vi "KR_Module.vi"() -> ()   [LabVIEW 2012]
doc: "SciScan 1.2 160630"
uses:
  Custom Control and Typedefs/ChannelSelector_for_PosSave.ctl
  Custom Control and Typedefs/Overlay Control.ctl
  Custom Control and Typedefs/UI Controls Refnum.ctl
  <vilib>/vision/Image Controls.llb/IMAQ Image.ctl
  SubVIs/Chnl_2_tab_Commands.ctl
  SubVIs/Image Validity FGV_Commands.ctl
  Custom Controls/MAIN Image panel tab Control type def.ctl
  CommonResource VIs/UI Control and Indicator properties_Commands.ctl
  Custom Control and Typedefs/ImageCluster.ctl
  GFG/GFG library.lvlib
  Libtiff3/libtiff3.llb/libtiff3.lvlib
panel:
  out "x-y":u32
  in  "Pop-Out 2":bool caption="Pop-Out"
  in  "Pop-Out":bool
  in  "no of grid lines 2":dbl(slide)=2.0 caption="Grid" min=0.0 step=1.0 scale=0.0..20.0
  in  "FOCUS2":bool
  in  "Overlay Controls":T1={"auto scale\n      Red "=TRUE, "Min Max Saved (Green)"={0.0, 1618.0}, "auto scale\n      Green"=TRUE, "Min Max Saved (Red)"={0.0, 1618.0}} {"Min Max Saved (Red)" scale=-32768.0..32767.0; "Min Max Saved (Green)" scale=-32768.0..32767.0}
  in  "File Path":path
  in  "Overlay":bool
  in  "Source":T2
  out "Saved Image":T3(plugin-control)
  out "Current Image":T3(plugin-control)
  # "Red (Current Image)"
  # "Green (Saved Image)"
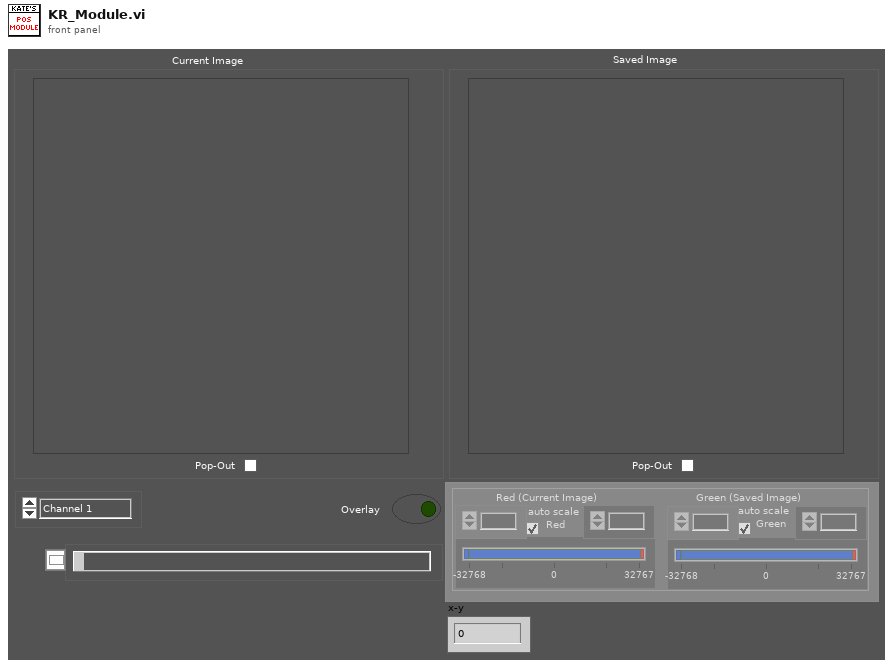
[diagram p1: front panel]
types:
  T1 = typedef "Overlay Control.ctl" = cluster{"auto scale\n      Red ":bool, "Min Max Saved (Green)":cluster{dbl, dbl}, "auto scale\n      Green":bool, "Min Max Saved (Red)":cluster{dbl, dbl}}
  T2 = typedef "ChannelSelector_for_PosSave.ctl" = enum16{"Channel 1", "Channel 2", "Channel 3", "Channel 4"}
  T3 = typedef "IMAQ Image.ctl" = refnum<image>
  T4 = typedef "Image Type" = u32
  T5 = typedef "UI Controls Refnum.ctl" = cluster{"GO TO":refnum<vi>, "Load List":refnum<vi>, "Big Table":refnum<vi>, "Notes Table":refnum<vi>, "New List":refnum<vi>, "Delete Item":refnum<vi>, "Set New Origin":refnum<vi>, "Set POI":refnum<vi>, "Saved Image":refnum<vi>, "Current Image":refnum<vi>, "step.size.xy 2":refnum<vi>, "step.size.z 2":refnum<vi>, "Source":refnum<vi>, "Table Up-End":refnum<vi>, "Table Up":refnum<vi>, "Table Down":refnum<vi>, "Table Down-End":refnum<vi>, "Copy Button":refnum<vi>, "Hide":refnum<vi>, "Overlay Controls":refnum<vi>, "Overlay":refnum<vi>, "XYGraph":refnum<vi>, "FOCUS2":refnum<vi>}
  T6 = enum8{"Enabled", "Disabled", "Disabled and Grayed Out"}
  T7 = typedef "ImageCluster.ctl" = cluster{"CurrentImage":T3, "SavedImage":T3}
  T8 = enum32{"Invalid", "Standard", "Closed", "Hidden", "Minimized", "Maximized"}
  T9 = typedef "Image Validity FGV_Commands.ctl" = enum16{"Set validity status", "Get Validity status"}
  T10 = typedef "Chnl_2_tab_Commands.ctl" = enum16{"ChannelToTab", "TabToChannel"}
  T11 = typedef "MAIN Image panel tab Control type def.ctl" = enum32{"Channel 1", "Channel 2", "Channel 3", "Channel 4", "all channels", "RGB overlay", "ROI", "arbitrary line scan"}
  T12 = typedef "UI Control and Indicator properties_Commands.ctl" = enum16{"Enable", "Disable", "Disable and Grey", "Make Visible", "Make Invisible"}
  T13 = cluster{"WaveformChartRef":refnum<vi>, "DigitalRef":refnum<vi>, "ArrayRef":refnum<vi>, "TabControlRef":refnum<vi>, "EnumRef":refnum<vi>, "RingRef":refnum<vi>, "BooleanRef":refnum<vi>, "KnobRef":refnum<vi>, "SlideRef":refnum<vi>, "PathRef":refnum<vi>, "StringRef":refnum<vi>, "ComboBox":refnum<vi>, "WaveformGraphRef":refnum<vi>}
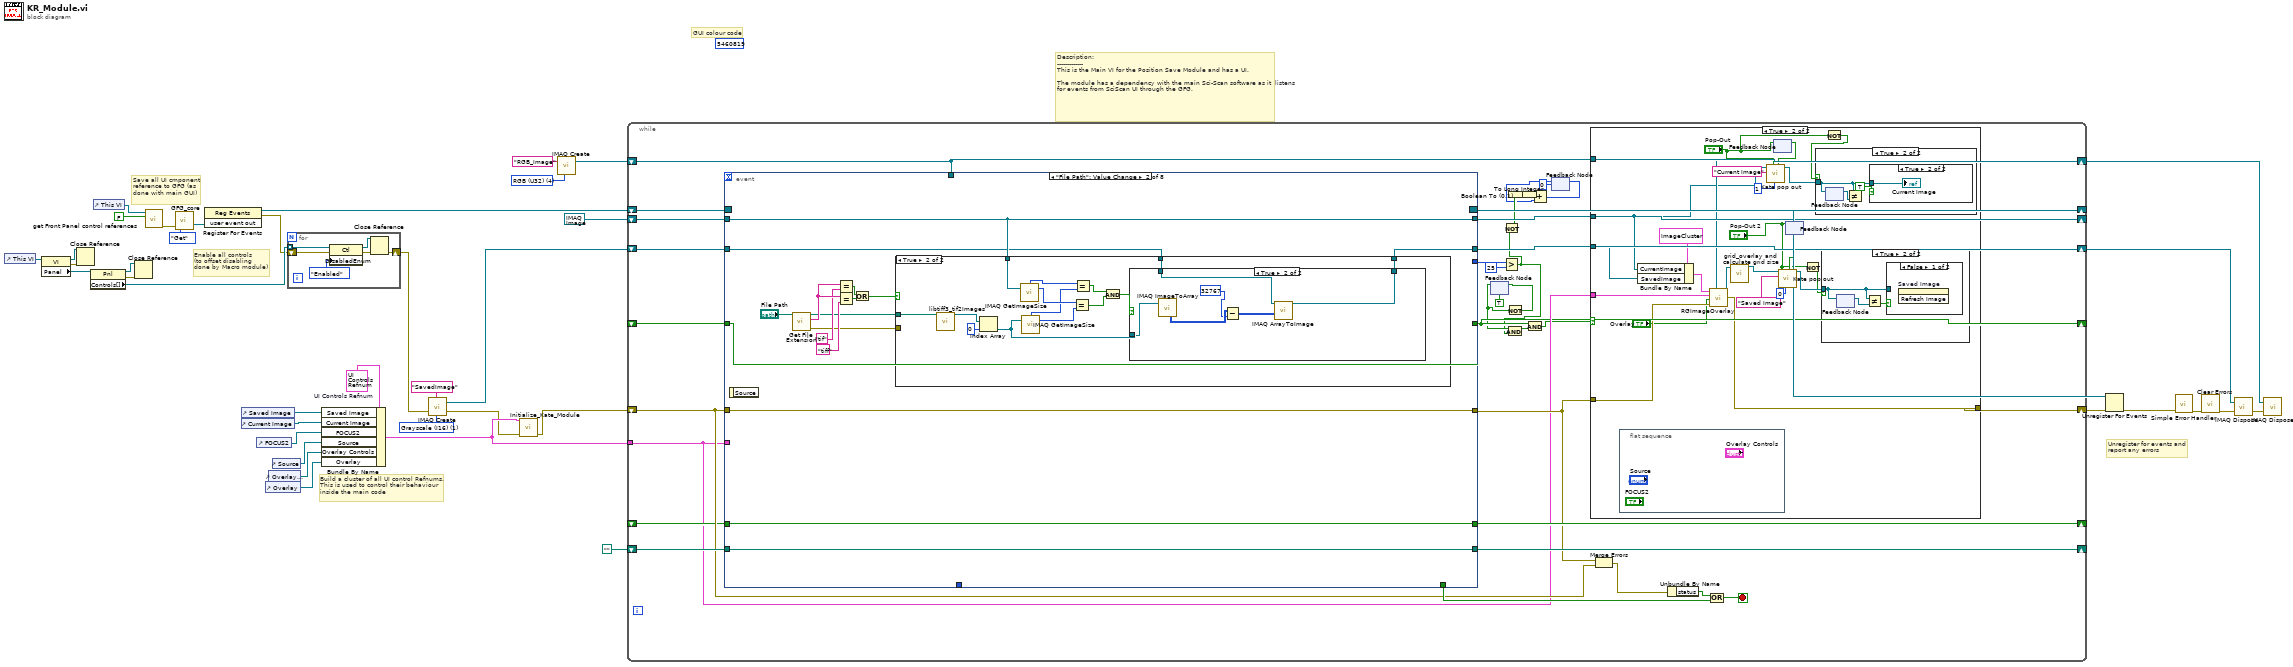
[diagram p0: block diagram]
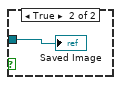
[diagram p4: hidden frame]
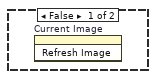
[diagram p6: hidden frame]
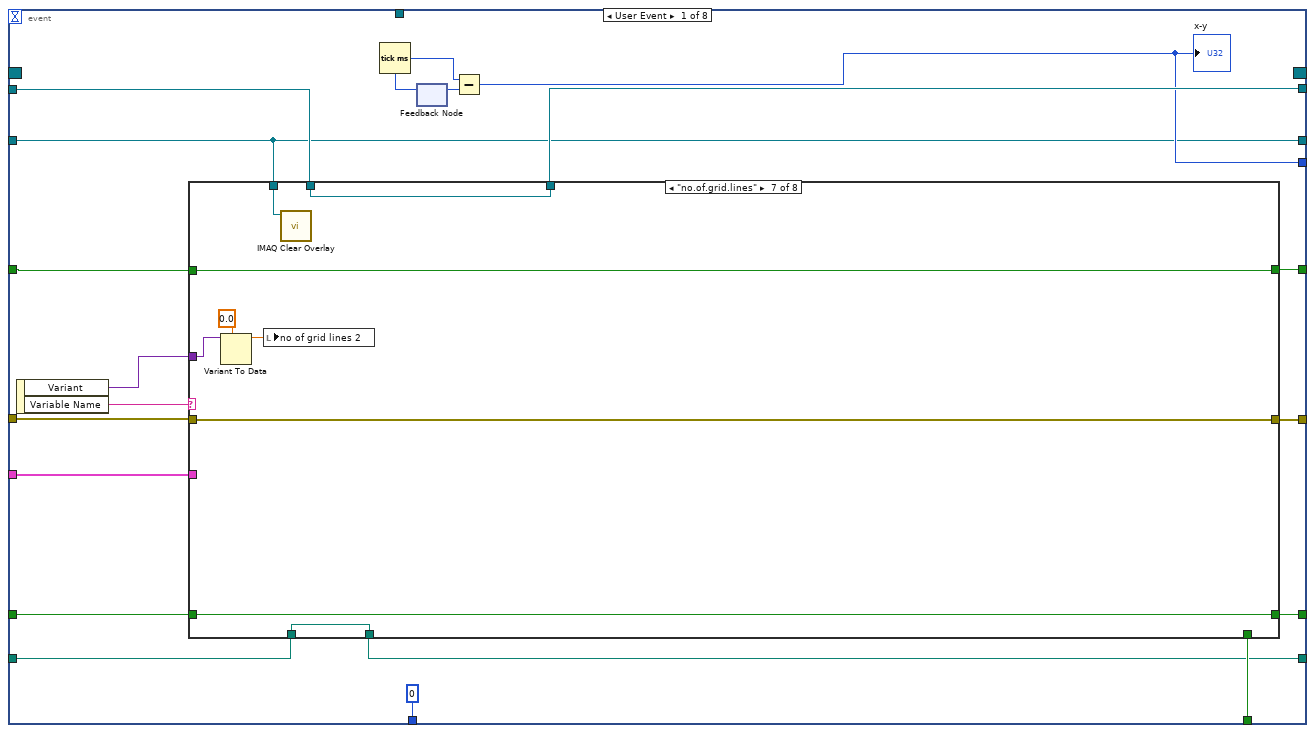
[diagram p7: hidden frame]
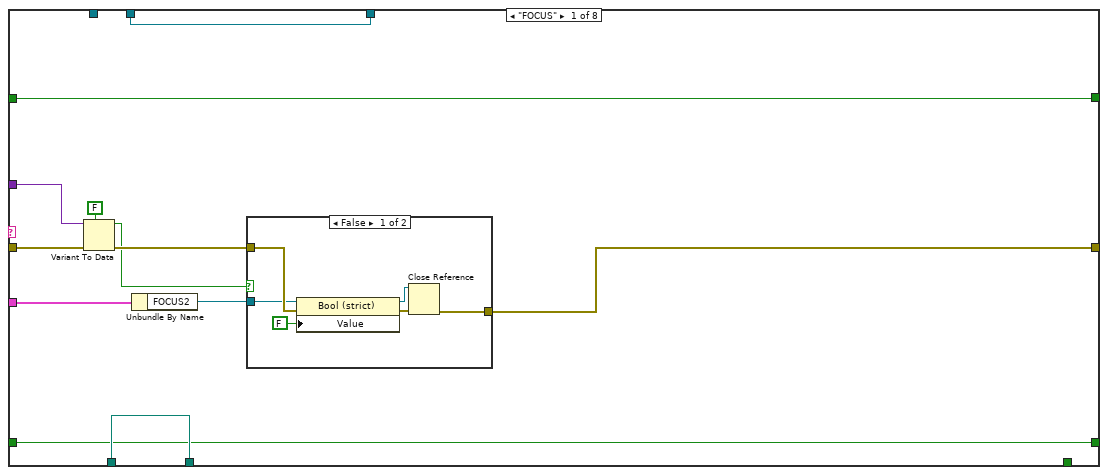
[diagram p8: hidden frame]
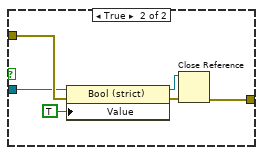
[diagram p9: hidden frame]
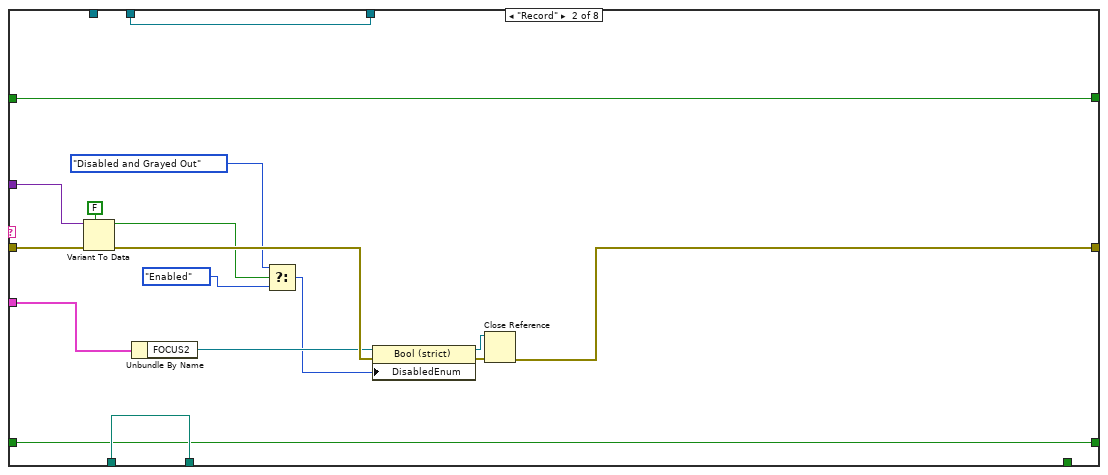
[diagram p10: hidden frame]
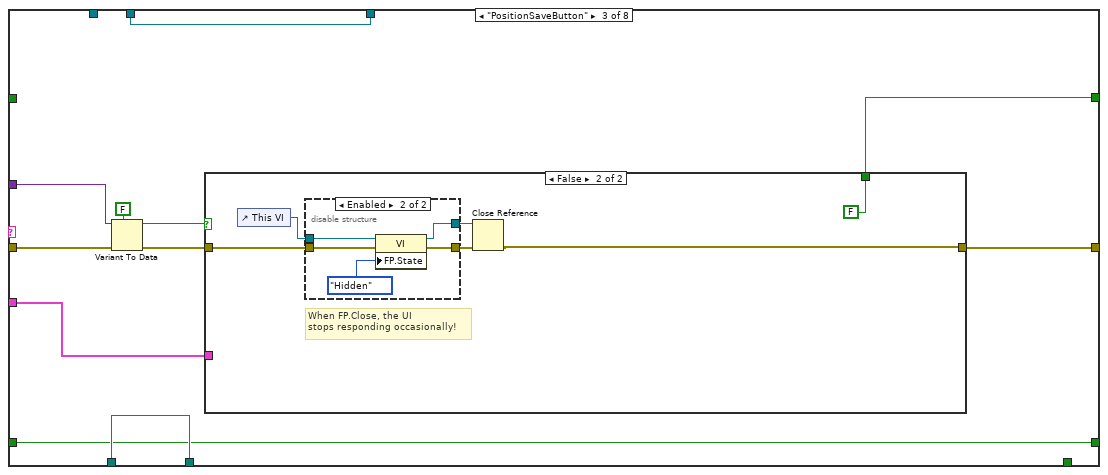
[diagram p11: hidden frame]
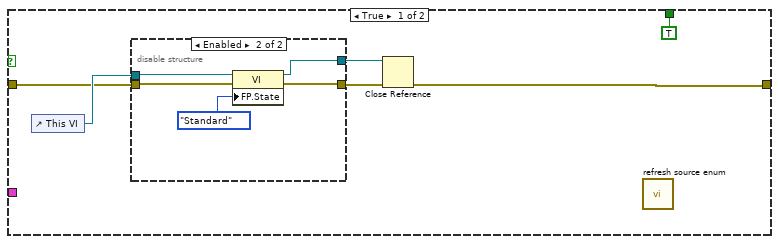
[diagram p12: hidden frame]
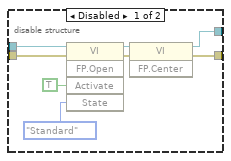
[diagram p13: hidden frame]
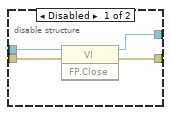
[diagram p14: hidden frame]
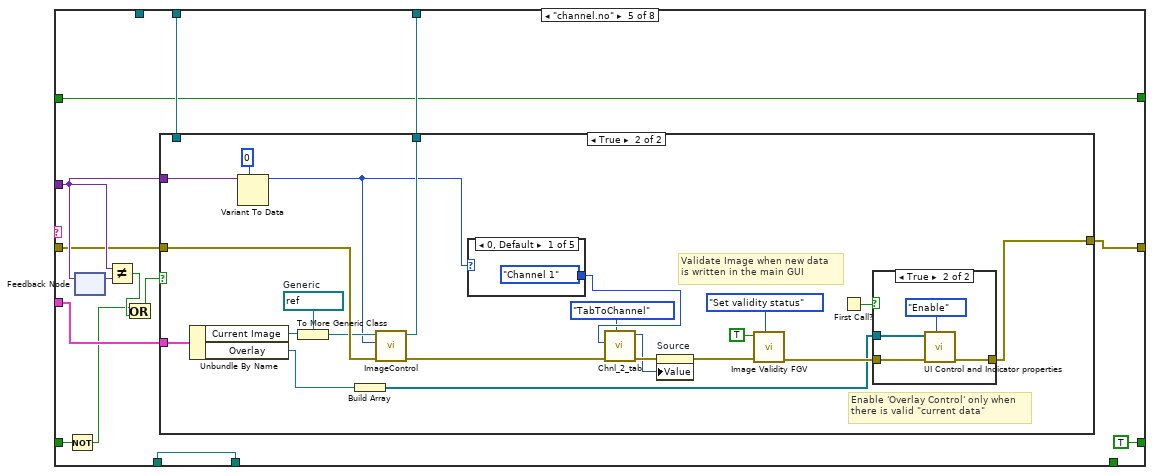
[diagram p16: hidden frame]
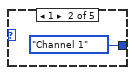
[diagram p18: hidden frame]
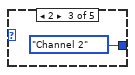
[diagram p19: hidden frame]
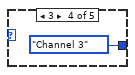
[diagram p20: hidden frame]
diagram:
  w25 = T4 4 items=["Grayscale (U8)", "Grayscale (I16)", "Grayscale (SGL)", "Complex (CSG)", "RGB (U32)", "HSL (U32)", "RGB (U64)", "Grayscale (U16)"] ("Image Type")
  w31 = T4 1 items=["Grayscale (U8)", "Grayscale (I16)", "Grayscale (SGL)", "Complex (CSG)", "RGB (U32)", "HSL (U32)", "RGB (U64)", "Grayscale (U16)"] ("Image Type")
  (unwired) u32 5460819 ("Active Cell:Cell Background Color")
  w37 = T5 {"GO TO"=refnum, "Load List"=refnum, "Big Table"=refnum, "Notes Table"=refnum, "New List"=refnum, "Delete Item"=refnum, "Set New Origin"=refnum, "Set POI"=refnum, "Saved Image"=refnum, "Current Image"=refnum, "step.size.xy 2"=refnum, "step.size.z 2"=refnum, "Source"=refnum, "Table Up-End"=refnum, "Table Up"=refnum, "Table Down"=refnum, "Table Down-End"=refnum, "Copy Button"=refnum, "Hide"=refnum, "Overlay Controls"=refnum, "Overlay"=refnum, "XYGraph"=refnum, "FOCUS2"=refnum}  # UI Controls Refnum
  # "Enable all controls\n(to offset disabling \ndone by Macro module)"
  # "GUI colour code"
  # "Save all UI cmponent reference to GFG (as done with main GUI)"
  # "Build a cluster of all UI control Refnums.\nThis is used to control their behaviour \ninside the main code"
  # "Unregister for events and \nreport any errors"
  # "Description:\n-------------\nThis is the Main VI for the Position Save Module and has a UI.\n\nThe module has a dependency with the main Sci-Scan software as it  listens for events from SciScan UI through the GFG."
  n1 = control-ref of="This VI"() -> (w17:refnum<vi>)
  n2 = property class="VI"(reference=w17) -> (reference out=w14:refnum<vi>, error out=w15:errorcluster, "Panel"=w16:refnum<vi>)  [unwired: 1 in]
  n3 = Close Reference(reference=w14, error in (no error)=w15) -> ()  [unwired: 1 out]
  n4 = property class="Pnl"(reference=w16) -> (reference out=w12:refnum<vi>, error out=w13:errorcluster, "Controls[]"=w11:refnum<vi>[])  [unwired: 1 in]
  n5 = control-ref of="This VI"() -> (w36:refnum<vi>)
  n6 = Close Reference(reference=w12, error in (no error)=w13) -> ()  [unwired: 1 out]
  n7 = call "get Front Panel control references.vi"("Signalling (Default: T)"=FALSE, "Main VI"=w36) -> ("error out"=w8:errorcluster)  [unwired: 9 in]
  n8 = call "GFG_core.vi"("error in (no error)"=w8, "Action"=enum16{"Init", "Set", "Get"}."Get") -> ("user event out"=w39:refnum<user-event>)  [unwired: 11 in, 6 out]
  n9 = register-events(w39) -> (reference out=w40:refnum<event-registration>, error out=w10:errorcluster)  [unwired: 2 in]
  n10 = control-ref of="Saved Image"() -> (w34:refnum<vi>)
  n11 = control-ref of="Current Image"() -> (w33:refnum<vi>)
  n12 = control-ref of="FOCUS2"() -> (w7:refnum<vi>)
  n13 = control-ref of="Overlay"() -> (w5:refnum<vi>)
  n14 = control-ref of="Overlay Controls"() -> (w4:refnum<vi>)
  n15 = control-ref of="Source"() -> (w6:refnum<vi>)
  n16 = for {
    tunnel: w11 -> [w47] mode=indexing
    shift-right: [w43] -> w9
    shift-left: w10 -> [w42]
    n17 = property class="Ctl"(reference=w47, error in=w42, "DisabledEnum"=T6."Enabled" ("Disabled")) -> (reference out=w44:refnum<vi>, error out=w45:errorcluster)
    n18 = Close Reference(reference=w44, error in (no error)=w45) -> (error out=w43:errorcluster)
  }
  n19 = Bundle By Name(cluster=w37, "Saved Image"=w34, "Current Image"=w33, "FOCUS2"=w7, "Source"=w6, "Overlay Controls"=w4, "Overlay"=w5) -> (w3:T5)
  n20 = call "IMAQ Create"("Image Name"="SavedImage", "Image Type"=w31, "error in (no error)"=w9) -> ("New Image"=w30:T3, "error out"=w2:errorcluster)  [unwired: 2 in]
  n21 = call "Initialize_Kate_Module.vi"("Error In"=w2, "UI Controls Refnum"=w3) -> ("Error Out"=w1:errorcluster)  [unwired: 9 in]
  n22 = call "IMAQ Create"("Image Name"="RGB_Image", "Image Type"=w25) -> ("New Image"=w24:T3)  [unwired: 3 in, 1 out]
  n23 = while {
    shift-right: [w67] -> w28
    shift-left: w1 -> [w74]
    shift-right: [w78] -> w38
    shift-left: w40 -> [w79]
    tunnel: w3 -> [w66]
    shift-right: [w64] -> _
    shift-left: T3 refnum ("Saved Image OUT") -> [w77]
    shift-right: [w72] -> w20
    shift-left: w30 -> [w76]
    shift-right: [w69] -> _
    shift-left: path "" -> [w75]
    shift-right: [w65] -> w19
    shift-left: w24 -> [w65]
    shift-right: [w71] -> _
    shift-left: _ -> [w70]
    shift-right: [w61] -> _
    shift-left: _ -> [w63]
    stop <- w80 stop-if-true
    n24 = event shown="[1] \"File Path\": Value Change" {
      selector: w79 -> [_ _ _ _ _ _ _ _]
      dyn-events: [_ _ _ _ _ _ _ _] -> w78
      timeout: _ -> [_ _ _ _ _ _ _ _]
      tunnel: [w133 _ _ _ _ _ _ _] -> w82
      tunnel: w74 -> [w132 w332 w362 w383 w403 w426 w448 w460]
      tunnel: [w131 w332 w361 w382 w403 w413 w445 w460] -> w68
      tunnel: w66 -> [w129 _ _ w385 _ _ _ _]
      tunnel: [w128 w329 w378 w389 w406 w423 w456 w463] -> w64
      tunnel: w77 -> [w125 w329 w378 w389 w406 w423 w456 w463]
      tunnel: [w115 w327 w377 w388 w405 w422 w455 w458] -> w72
      tunnel: w76 -> [w115 w328 w377 w388 w405 w422 w455 w462]
      tunnel: [w126 w331 w375 w387 w404 w418 w454 w459] -> w69
      tunnel: w75 -> [w127 w331 w375 w387 w404 w418 w454 w459]
      tunnel: [0 ("x-y 2") _ _ 1 ("x-y 2") 2 ("x-y 2") 17 ("x-y 2") 19 ("x-y 2") _] -> _
      tunnel: [w122 w330 w360 w380 w401 w408 w443 w461] -> w71
      tunnel: w70 -> [w121 w330 w360 w380 w401 w408 w443 w461]
      tunnel: w65 -> [_ _ _ _ _ _ _ _]
      tunnel: [w120 w326 w359 w379 w400 w407 w442 w457] -> w61
      tunnel: w63 -> [w119 w326 w359 w379 w400 w407 w442 w457]
      tunnel: [w116 _ _ _ _ _ _ _] -> w56
      event User Event {
        n25 = event-data() -> ("Variant"=w130:variant, "Variable Name"=w123:string)  [unwired: 1 in]
        n26 = case shown="\"no.of.grid.lines\"" w123 {
          tunnel: [_ _ _ _ _ _ _ TRUE] -> w133
          tunnel: w132 -> [w142 w171 w185 w222 w235 w284 w307 w312]
          tunnel: [w138 w168 w180 w222 w232 w281 w307 w312] -> w131
          tunnel: w130 -> [w140 w169 w183 _ w237 w287 w306 _]
          tunnel: [w144 w173 w177 w224 w234 w285 w310 w315] -> w128
          tunnel: w129 -> [w137 w167 w178 _ w233 w283 _ _]
          tunnel: w127 -> [w145 w174 w179 w223 w238 w286 w309 _]
          tunnel: [w145 w174 w179 w223 w238 w286 w309 path ""] -> w126
          tunnel: w125 -> [w144 w173 w177 w224 w226 w285 w310 w315]
          tunnel: [w135 w165 w176 w221 TRUE ("Validity status IN") w274 w308 w314] -> w122
          tunnel: w121 -> [w135 w165 w176 w221 w228 w274 w308 w314]
          tunnel: [w134 w158 w175 w220 w225 w273 w303 w311] -> w120
          tunnel: w119 -> [w134 w158 _ w220 w225 w273 w303 w311]
          tunnel: w115 -> [_ _ _ _ _ _ w302 _]
          frame "FOCUS" {
            n27 = Variant To Data(error in=w142, type=FALSE ("Value"), Variant=w140) -> (data=w139:bool, error out=w141:errorcluster)
            n28 = Unbundle By Name(w137) -> ("FOCUS2"=w136:refnum<vi>)
            n29 = case shown="False" w139 {
              tunnel: w141 -> [w150 w156]
              tunnel: [w147 w153] -> w138
              tunnel: w136 -> [w146 w152]
              frame False {
                n30 = property class="Bool (strict)"(reference=w146, error in=w150, "Value"=FALSE) -> (reference out=w148:refnum<vi>, error out=w149:errorcluster)
                n31 = Close Reference(reference=w148, error in (no error)=w149) -> (error out=w147:errorcluster)
              }
              frame True {
                n32 = property class="Bool (strict)"(reference=w152, error in=w156, "Value"=TRUE) -> (reference out=w154:refnum<vi>, error out=w155:errorcluster)
                n33 = Close Reference(reference=w154, error in (no error)=w155) -> (error out=w153:errorcluster)
              }
            }
          }
          frame "Record" {
            n34 = Variant To Data(error in=w171, type=FALSE ("Value"), Variant=w169) -> (data=w164:bool, error out=w170:errorcluster)
            n35 = Unbundle By Name(w167) -> ("FOCUS2"=w166:refnum<vi>)
            n36 = Select(t=T6."Disabled and Grayed Out" ("Disabled"), s=w164, f=T6."Enabled" ("Disabled")) -> (s? t:f=w159:T6)
            n37 = property class="Bool (strict)"(reference=w166, error in=w170, "DisabledEnum"=w159) -> (reference out=w162:refnum<vi>, error out=w163:errorcluster)
            n38 = Close Reference(reference=w162, error in (no error)=w163) -> (error out=w168:errorcluster)
          }
          frame "PositionSaveButton" {
            n39 = Variant To Data(error in=w185, type=FALSE, Variant=w183) -> (data=w181:bool, error out=w182:errorcluster)
            n40 = case shown="False" w181 {
              tunnel: w182 -> [w190 w209]
              tunnel: [w187 w206] -> w180
              tunnel: w178 -> [_ _]
              tunnel: [TRUE FALSE] -> w175
              frame True {
                n41 = control-ref of="This VI"() -> (w191:refnum<vi>)
                n42 = disable-structure shown="Enabled" {
                  disable-tunnel: w191 -> [w199 w203]
                  disable-tunnel: w190 -> [w198 w202]
                  disable-tunnel: [w193 w201] -> w189
                  disable-tunnel: [w192 w200] -> w188
                  frame Disabled {
                    n43 = invoke class="VI" method="FP.Open"(reference=w199, error in=w198, "Activate"=TRUE ("Activate?"), "State"=T8."Standard") -> (reference out=w195:refnum<vi>, error out=w194:errorcluster)  [unwired: 1 in, 3 out]
                    n44 = invoke class="VI" method="FP.Center"(reference=w195, error in=w194) -> (reference out=w192:refnum<vi>, error out=w193:errorcluster)  [unwired: 1 in, 1 out]
                  }
                  frame Enabled {
                    n45 = property class="VI"(reference=w203, error in=w202, "FP.State"=T8."Standard" ("Front Panel Window:State")) -> (reference out=w200:refnum<vi>, error out=w201:errorcluster)
                  }
                }
                n46 = Close Reference(reference=w188, error in (no error)=w189) -> (error out=w187:errorcluster)
                n47 = call "refresh source enum.vi"() -> ()  [unwired: 12 in]
              }
              frame False {
                # "When FP.Close, the UI\nstops responding occasionally!"
                n48 = control-ref of="This VI"() -> (w210:refnum<vi>)
                n49 = disable-structure shown="Enabled" {
                  disable-tunnel: w210 -> [w214 w217]
                  disable-tunnel: w209 -> [w213 w218]
                  disable-tunnel: [w212 w219] -> w208
                  disable-tunnel: [w211 w215] -> w207
                  frame Disabled {
                    n50 = invoke class="VI" method="FP.Close"(reference=w214, error in=w213) -> (reference out=w211:refnum<vi>, error out=w212:errorcluster)  [unwired: 1 in, 1 out]
                  }
                  frame Enabled {
                    n51 = property class="VI"(reference=w217, error in=w218, "FP.State"=T8."Hidden" ("Front Panel Window:State")) -> (reference out=w215:refnum<vi>, error out=w219:errorcluster)
                  }
                }
                n52 = Close Reference(reference=w207, error in (no error)=w208) -> (error out=w206:errorcluster)
              }
            }
          }
          frame Default {
          }
          frame "channel.no" {
            n53 = Not(x=w228) -> (.not. x?=w227:bool)
            n54 = feedback #1() -> (w236:variant)  [unwired: 1 in]
            n55 = feedback-in #1(w237) -> ()
            n56 = Not Equal?(x=w237, y=w236) -> (x != y?=w230:bool)
            n57 = Or(x=w227, y=w230) -> (x .or. y?=w229:bool)
            n58 = case shown="True" w229 {
              tunnel: w237 -> [_ w262]
              tunnel: w235 -> [w239 w261]
              tunnel: [w240 w260] -> w234
              tunnel: w233 -> [_ w259]
              tunnel: [w239 w258] -> w232
              tunnel: w226 -> [w240 _]
              frame False {
              }
              frame True {
                w248 = refnum<vi> refnum  # Generic
                # "Enable 'Overlay Control' only when there is valid \"current data\""
                # "Validate Image when new data\nis written in the main GUI"
                n59 = Unbundle By Name(w259) -> ("Current Image"=w251:refnum<vi>, "Overlay"=w250:refnum<vi>)
                n60 = Variant To Data(type=0, Variant=w262) -> (data=w247:i32)  [unwired: 1 in, 1 out]
                n61 = To More Generic Class(target class=w248, reference=w251) -> (generic class reference=w252:refnum<vi>)
                n62 = Build Array(w250) -> (w249:refnum<vi>[])
                n63 = call "ImageControl.vi"("Error In"=w261, "Channel No"=w247, "Image Refnum (Generic)"=w252) -> ("Error Out"=w253:errorcluster, "Current Image"=w260:T3)  [unwired: 7 in]
                n64 = case shown="0, Default" w247 {
                  tunnel: [MAIN_Image_panel_tab_Control_type_def."Channel 1" ("Tab IN") MAIN_Image_panel_tab_Control_type_def."Channel 1" ("Tab IN") MAIN_Image_panel_tab_Control_type_def."Channel 2" ("Tab IN") MAIN_Image_panel_tab_Control_type_def."Channel 3" ("Tab IN") MAIN_Image_panel_tab_Control_type_def."Channel 4" ("Tab IN")] -> w245
                  frame 0, Default {
                  }
                  frame 1 {
                  }
                  frame 2 {
                  }
                  frame 3 {
                  }
                  frame 4 {
                  }
                }
                n65 = call "Chnl_2_tab.vi"("Command"=Chnl_2_tab_Commands."TabToChannel", "Error In"=w253, "Tab IN"=w245) -> ("Error Out"=w255:errorcluster, "Channel  OUT"=w254:T2)  [unwired: 6 in, 1 out]
                n66 = property on="Source" class="Enum (strict)"(error in=w255, "Value"=w254) -> (error out=w256:errorcluster)  [unwired: 1 in, 1 out]
                n67 = call "Image Validity FGV.vi"("Image Validity FGV_Commands"=Image_Validity_FGV_Commands."Set validity status", "Error In"=w256, "Validity status IN"=TRUE) -> ("Error Out"=w257:errorcluster)  [unwired: 7 in, 1 out]
                n68 = First Call?() -> (First Call?: T/F=w241:bool)
                n69 = case shown="True" w241 {
                  tunnel: w257 -> [w268 w271]
                  tunnel: [w268 w270] -> w258
                  tunnel: w249 -> [_ w269]
                  frame False {
                  }
                  frame True {
                    n70 = call "UI Control and Indicator properties.vi"("Enable Command"=UI_Control_and_Indicator_properties_Commands."Enable", "Error In"=w271, "Control Refnums"=w269) -> ("Error Out"=w270:errorcluster)  [unwired: 8 in]
                  }
                }
              }
            }
          }
          frame "MAIN.Image.panels.", "MAIN.Image.panels.reso." {
            # "Clear Error  91 if it occurs. Eg. when \nGFG variable for the 'main image panel' of the wrong  type is set - This is triggered by MACRO MODULE"
            n71 = Unbundle By Name(w283) -> ("Source"=w282:refnum<vi>)
            n72 = Variant To Data(error in=w284, type=0, Variant=w287) -> (data=w279:i32, error out=w277:errorcluster)
            n73 = call "Clear Specific Errors.vi"("Error In"=w277, "Error number In"=91) -> ("Error Out"=w276:errorcluster, "Error Cleared?"=w275:bool)  [unwired: 8 in]
            n74 = case shown="True" w275 {
              tunnel: w282 -> [w293 _]
              tunnel: [w292 w301] -> w281
              tunnel: w279 -> [w290 _]
              tunnel: w276 -> [w288 w301]
              frame False {
                n75 = Less?(x=w290, y=4) -> (x < y?=w291:bool)
                n76 = case shown="True" w291 {
                  tunnel: w293 -> [_ w300]
                  tunnel: [w294 w297] -> w292
                  tunnel: w290 -> [_ w296]
                  tunnel: w288 -> [w294 w295]
                  frame False {
                  }
                  frame True {
                    n77 = property class="Enum (strict)"(reference=w300, error in=w295, "Value"=w296) -> (reference out=w298:refnum<vi>, error out=w299:errorcluster)
                    n78 = Close Reference(reference=w298, error in (no error)=w299) -> (error out=w297:errorcluster)
                  }
                }
              }
              frame True {
                # "Error 91 has been cleared.\nWrong 'Image Panels GFG variable' set.\nDO NOTHING!"
              }
            }
          }
          frame "no.of.grid.lines" {
            n79 = Variant To Data(type=0.0 ("no of grid lines 2"), Variant=w306) -> (data=w304:dbl)  [unwired: 1 in, 1 out]
            n80 = local write "no of grid lines 2"(w304) -> ()
            n81 = call "IMAQ Clear Overlay"("Image"=w302) -> ()  [unwired: 9 in, 2 out]
          }
          frame "QUIT" {
          }
        }
        n82 = Tick Count (ms)() -> (millisecond timer value=w118:u32)
        n83 = feedback-in #2(w118) -> ()
        n84 = feedback #2() -> (w117:u32)  [unwired: 1 in]
        n85 = Subtract(x=w118, y=w117) -> (x-y=w116:u32)
        "x-y" <- w116
      }
      event "File Path": Value Change {
        n86 = event-data() -> ()  [unwired: 1 in, 1 out]
        n87 = call <vilib>:"Get File Extension.vi"("file"="File Path") -> ("error out"=w317:errorcluster, "lowercase file extension"=w325:string, "dup file"=w318:path)  [unwired: 7 in, 1 out]
        n88 = Equal?(x=w325, y="tif") -> (x = y?=w322:bool)
        n89 = Equal?(x=w325, y="tiff") -> (x = y?=w321:bool)
        n90 = Or(x=w322, y=w321) -> (x .or. y?=w319:bool)
        n91 = case shown="True" w319 {
          tunnel: w329 -> [_ w350]
          tunnel: w328 -> [w333 w342]
          tunnel: [w333 w341] -> w327
          tunnel: w318 -> [_ w338]
          tunnel: w317 -> [w335 _]
          frame False {
            # "Ignore this file, as it's not a TIFF."
            n92 = property on="File Path" class="Path"(error in=w335, "Value"=path "" ("File Path")) -> ()  [unwired: 1 in, 2 out]
            n93 = One Button Dialog(message="Invalid file format! Please select a TIFF file and try again.") -> ()  [unwired: 1 in, 1 out]
          }
          frame True {
            n94 = call "libtiff3_tif2Images.vi"("Input path"=w338) -> ("ImageArray"=w340:T3[])  [unwired: 9 in, 1 out]
            n95 = Index Array(array=w340, index=0) -> (element=w337:T3)
            n96 = call "IMAQ GetImageSize"("Image"=w350) -> ("Y Resolution"=w349:i32, "X Resolution"=w346:i32)  [unwired: 3 in, 1 out]
            n97 = call "IMAQ GetImageSize"("Image"=w337) -> ("Y Resolution"=w348:i32, "X Resolution"=w347:i32)  [unwired: 3 in, 1 out]
            n98 = Equal?(x=w349, y=w348) -> (x = y?=w344:bool)
            n99 = Equal?(x=w346, y=w347) -> (x = y?=w345:bool)
            n100 = And(x=w345, y=w344) -> (x .and. y?=w343:bool)
            n101 = case shown="True" w343 {
              tunnel: w337 -> [_ w358]
              tunnel: w342 -> [w352 w354]
              tunnel: [w352 w353] -> w341
              frame False {
                n102 = One Button Dialog(message="Image Size Mismatch") -> ()  [unwired: 1 in, 1 out]
              }
              frame True {
                n103 = call "IMAQ ImageToArray"("Image"=w358) -> ("Image Pixels (U16)"=w357:u16[][])  [unwired: 3 in, 4 out]
                n104 = Subtract(x=w357, y=i16 32767) -> (x-y=w355:u16[][])
                n105 = call "IMAQ ArrayToImage"("Image Pixels (I16)"=w355, "Image"=w354) -> ("Image Out"=w353:T3)  [unwired: 8 in, 1 out]
              }
            }
          }
        }
      }
      event Panel Close? {
        n106 = event-data() -> ()  [unwired: 1 in, 1 out]
        n107 = control-ref of="This VI"() -> (w374:refnum<vi>)
        n108 = property class="VI"(reference=w374, error in=w362, "FP.State"=T8."Hidden" ("Front Panel Window:State")) -> (reference out=w372:refnum<vi>, error out=w373:errorcluster)
        n109 = Close Reference(reference=w372, error in (no error)=w373) -> (error out=w365:errorcluster)
        n110 = call "GFGfpRefGet.vi"("error in (no error)"=w365, "Variable Name in"="PositionSaveButton") -> ("error out"=w369:errorcluster, "output cluster"=w370:T13)  [unwired: 8 in]
        n111 = Unbundle By Name(w370) -> ("BooleanRef"=w368:refnum<vi>)
        n112 = property class="Bool"(reference=w368, error in=w369, "Value"=FALSE) -> (reference out=w366:refnum<vi>, error out=w367:errorcluster)
        n113 = Close Reference(reference=w366, error in (no error)=w367) -> (error out=w361:errorcluster)
        n114 = event-data("Discard?"=TRUE) -> ()  [unwired: 1 in, 1 out]
      }
      event "Overlay": Value Change {
        # "Enable/Disable the Overlay cluster according to\nthe value"
        n115 = event-data() -> ("NewVal"=w386:bool)  [unwired: 1 in]
        n116 = Unbundle By Name(w385) -> ("Overlay Controls"=w384:refnum<vi>)
        n117 = case shown="False" w386 {
          tunnel: w384 -> [w392 w397]
          tunnel: w383 -> [w393 w398]
          tunnel: [w390 w395] -> w382
          frame True {
            n118 = Build Array(w392) -> (w391:refnum<vi>[])
            n119 = call "UI Control and Indicator properties.vi"("Enable Command"=UI_Control_and_Indicator_properties_Commands."Enable", "Error In"=w393, "Control Refnums"=w391) -> ("Error Out"=w390:errorcluster)  [unwired: 8 in]
          }
          frame False {
            n120 = Build Array(w397) -> (w396:refnum<vi>[])
            n121 = call "UI Control and Indicator properties.vi"("Enable Command"=UI_Control_and_Indicator_properties_Commands."Disable and Grey", "Error In"=w398, "Control Refnums"=w396) -> ("Error Out"=w395:errorcluster)  [unwired: 8 in]
          }
        }
      }
      event Value Change {
        # "Make sure the loop executes, to update the Image whenever there is a change in  any of the Overlay controls"
        n122 = event-data() -> ()  [unwired: 1 in, 1 out]
      }
      event Value Change {
        # "Set the Main Image panel\n(EITHER reso or galvo), depending on\nthe system in use"
        # "Typecast to int to make it compatible\nwith both tab types (galvo and reso)"
        # "On user selecting a different channel,\nset the channel no variable to trigger\nthe user event case which refreshes\ncurrent data"
        n123 = event-data() -> ("NewVal"=w424:T2)  [unwired: 1 in]
        n124 = call "Chnl_2_tab.vi"("Command"=Chnl_2_tab_Commands."ChannelToTab", "Error In"=w426, "Channel IN"=w424) -> ("Error Out"=w425:errorcluster, "Tab Out"=w416:T11)  [unwired: 6 in, 1 out]
        n125 = Type Cast(type=0 ("x-y 2"), x=w416) -> (*(type *) &x=w409:i32)
        n126 = Increment(x=w409) -> (x+1=w410:i32)
        n127 = Build Array("MAIN Image panels " ("Variable Name in"), "MAIN Image panels reso " ("Variable Name in")) -> (w419:string[])
        n128 = for {
          tunnel: w409 -> [w435]
          tunnel: w419 -> [w432] mode=indexing
          shift-right: [w434] -> w414
          shift-left: w425 -> [w433]
          n129 = call "GFG_core.vi"("Variable Name in"=w432, "error in (no error)"=w433) -> ("Variant Out"=w431:variant, "error out"=w428:errorcluster)  [unwired: 11 in, 5 out]
          n130 = Not Equal?(x=variant, y=w431) -> (x != y?=w429:bool)
          n131 = case shown="True" w429 {
            tunnel: w435 -> [_ w440]
            tunnel: [w436 w439] -> w434
            tunnel: w432 -> [_ w438]
            tunnel: w428 -> [w436 w437]
            frame False {
            }
            frame True {
              n132 = call "GFG_core.vi"("Variable Name in"=w438, "Variant in"=w440, "error in (no error)"=w437, "Action"=enum16{"Init", "Set", "Get"}."Set") -> ("error out"=w439:errorcluster)  [unwired: 9 in, 6 out]
            }
          }
        }
        n133 = call "GFG_core.vi"("Variable Name in"="channel.no", "Variant in"=w410, "error in (no error)"=w414, "Action"=enum16{"Init", "Set", "Get"}."Set") -> ("error out"=w413:errorcluster)  [unwired: 9 in, 6 out]
      }
      event "FOCUS2": Value Change {
        n134 = event-data() -> ("NewVal"=w449:bool)  [unwired: 1 in]
        n135 = To Variant(anything=w449) -> (Variant=w450:variant)
        n136 = call "GFGfpRefGet.vi"("Variable Name in"="FOCUS") -> ("output cluster"=w452:T13)  [unwired: 9 in, 1 out]
        n137 = Unbundle By Name(w452) -> ("BooleanRef"=w451:refnum<vi>)
        n138 = property class="Bool"(reference=w451, error in=w448, "Val(Sgnl)"=w450) -> (reference out=w446:refnum<vi>, error out=w447:errorcluster)
        n139 = Close Reference(reference=w446, error in (no error)=w447) -> (error out=w445:errorcluster)
      }
      event "no of grid lines 2": Value Change {
        n140 = event-data() -> ()  [unwired: 1 in, 1 out]
        n141 = disable-structure shown="Disabled" {
          frame Disabled {
            n142 = call "GFG_core.vi"("Variable Name in"="no of grid lines", "Variant in"="no of grid lines 2", "Action"=enum16{"Init", "Set", "Get", "Clear"}."Set") -> ()  [unwired: 10 in, 7 out]
          }
          frame Enabled {
          }
        }
        n143 = call "IMAQ Clear Overlay"("Image"=w462) -> ("Image Out"=w458:T3)  [unwired: 9 in, 1 out]
      }
    }
    n144 = feedback #3(TRUE) -> (w59:bool)
    n145 = Greater?(x=w56, y=u32 25) -> (0:w54:bool)
    n146 = Not(x=w54) -> (.not. x?=w53:bool)
    n147 = And(x=w59, y=w54) -> (x .and. y?=w57:bool)
    n148 = Boolean To (0,1)(Boolean=w53) -> (0, 1=w52:i16)
    n149 = Not(x=w59) -> (.not. x?=w58:bool)
    n150 = feedback-in #3(w58) -> ()
    n151 = To Long Integer(number=w52) -> (32bit integer=w51:i32)
    n152 = And(x=w61, y=w57) -> (x .and. y?=w60:bool)
    n153 = feedback #4(0) -> (w49:i32)
    n154 = Add(x=w51, y=w49) -> (x+y=w50:i32)
    n155 = feedback-in #4(w50) -> ()
    n156 = case shown="True" w60 {
      tunnel: w72 -> [_ w105]
      tunnel: w68 -> [w83 w104]
      tunnel: [w83 w103] -> w67
      tunnel: w66 -> [_ w102]
      tunnel: w65 -> [_ w98]
      tunnel: w64 -> [_ w94]
      frame False {
      }
      frame True {
        n157 = flat-sequence {
          frame #0 {
          }
        }
        n158 = Bundle By Name(cluster=T7 {"CurrentImage"=refnum, "SavedImage"=refnum} ("Image Input Cluster"), "CurrentImage"=w94, "SavedImage"=w105) -> (w101:T7)
        n159 = call "RGImageOverlay.vi"("RGB_Image"=w98, "Error In"=w104, "Overlay?"="Overlay", "UI Controls Refnum"=w102, "Image Input Cluster"=w101) -> ("Error Out"=w103:errorcluster, "Saved Image"=w100:T3)  [unwired: 5 in]
        n160 = call "grid_overlay and calculate grid size.vi"("Image In"=w100) -> ("Image Out"=w97:T3)  [unwired: 10 in]
        n161 = feedback #5() -> (w91:bool)  [unwired: 1 in]
        n162 = call "Kate pop out.vi"("prev iteration"=w91, "Window Number (0...15)"=1, "pop out"="Pop-Out", "Title"="Current Image", "Image"=w94) -> ("Image Out (duplicate)"=w89:T3)  [unwired: 6 in]
        n163 = feedback-in #5("Pop-Out") -> ()
        n164 = feedback #6() -> (w90:bool)  [unwired: 1 in]
        n165 = call "Kate pop out.vi"("prev iteration"=w90, "Window Number (0...15)"=0, "pop out"="Pop-Out 2", "Title"="Saved Image", "Image"=w97) -> ("Image Out (duplicate)"=w88:T3)  [unwired: 6 in]
        n166 = feedback-in #6("Pop-Out 2") -> ()
        n167 = Not(x="Pop-Out 2") -> (.not. x?=w84:bool)
        n168 = case shown="True" w84 {
          tunnel: w88 -> [_ w108]
          frame False {
          }
          frame True {
            n169 = feedback #7() -> (w109:T3)  [unwired: 1 in]
            n170 = feedback-in #7(w108) -> ()
            n171 = Not Equal?(x=w108, y=w109) -> (x != y?=w107:bool)
            n172 = case shown="False" w107 {
              tunnel: w108 -> [_ w110]
              frame False {
                n173 = invoke on="Saved Image" class="ImageControl" method="Refresh Image"() -> ()  [unwired: 3 in, 3 out]
              }
              frame True {
                "Saved Image" <- w110
              }
            }
          }
        }
        n174 = Not(x="Pop-Out") -> (.not. x?=w86:bool)
        n175 = case shown="True" w86 {
          tunnel: w89 -> [_ w112]
          frame False {
          }
          frame True {
            n176 = feedback #8() -> (w113:T3)  [unwired: 1 in]
            n177 = feedback-in #8(w112) -> ()
            n178 = Not Equal?(x=w112, y=w113) -> ()  [unwired: 1 out]
            n179 = case shown="True" TRUE {
              tunnel: w112 -> [_ w114]
              frame False {
                n180 = invoke on="Current Image" class="ImageControl" method="Refresh Image"() -> ()  [unwired: 3 in, 3 out]
              }
              frame True {
                "Current Image" <- w114
              }
            }
          }
        }
      }
    }
    n181 = Merge Errors(w68, w74) -> (w73:errorcluster)
    n182 = Unbundle By Name(w73) -> ("status"=w81:bool)
    n183 = Or(x=w81, y=w82) -> (x .or. y?=w80:bool)
  }
  n184 = Unregister For Events(event registration refnum=w38, error in=w28) -> (error out=w41:errorcluster)
  n185 = call <vilib>:"Simple Error Handler.vi"("error in (no error)"=w41) -> ("error out"=w29:errorcluster)  [unwired: 4 in, 4 out]
  n186 = call <vilib>:"Clear Errors.vi"("error in (no error)"=w29) -> ("error out"=w21:errorcluster)  [unwired: 6 in]
  n187 = call "IMAQ Dispose"("Image"=w20, "error in (no error)"=w21) -> ("error out"=w18:errorcluster)  [unwired: 4 in]
  n188 = call "IMAQ Dispose"("Image"=w19, "error in (no error)"=w18) -> ()  [unwired: 4 in, 1 out]
